vi "WSVCAP SHL Host LL I2C Build and Parse Read Message.vi"(0 "C1 Read Data In":u8[][](array[numeric]) format="%.0x", 1 "Message In":string, 5 "C2 Read Data":u8[][](array[numeric]) format="%.0x", 7 "C3 Read Data":u8[][](array[numeric]) format="%.0x", 9 "Status In":u8[](array[numeric]), 11 "error in":errorcluster) -> (3 "Message Out":string, 4 "C1 Read Data Out":u8[][](array[numeric]) format="%.0x", 6 "C2 Read Data Out":u8[][](array[numeric]) format="%.0x", 8 "C3 Read Data Out":u8[][](array[numeric]) format="%.0x", 10 "Status":u8[](array[numeric]), 15 "error out":errorcluster)   [LabVIEW 2012]
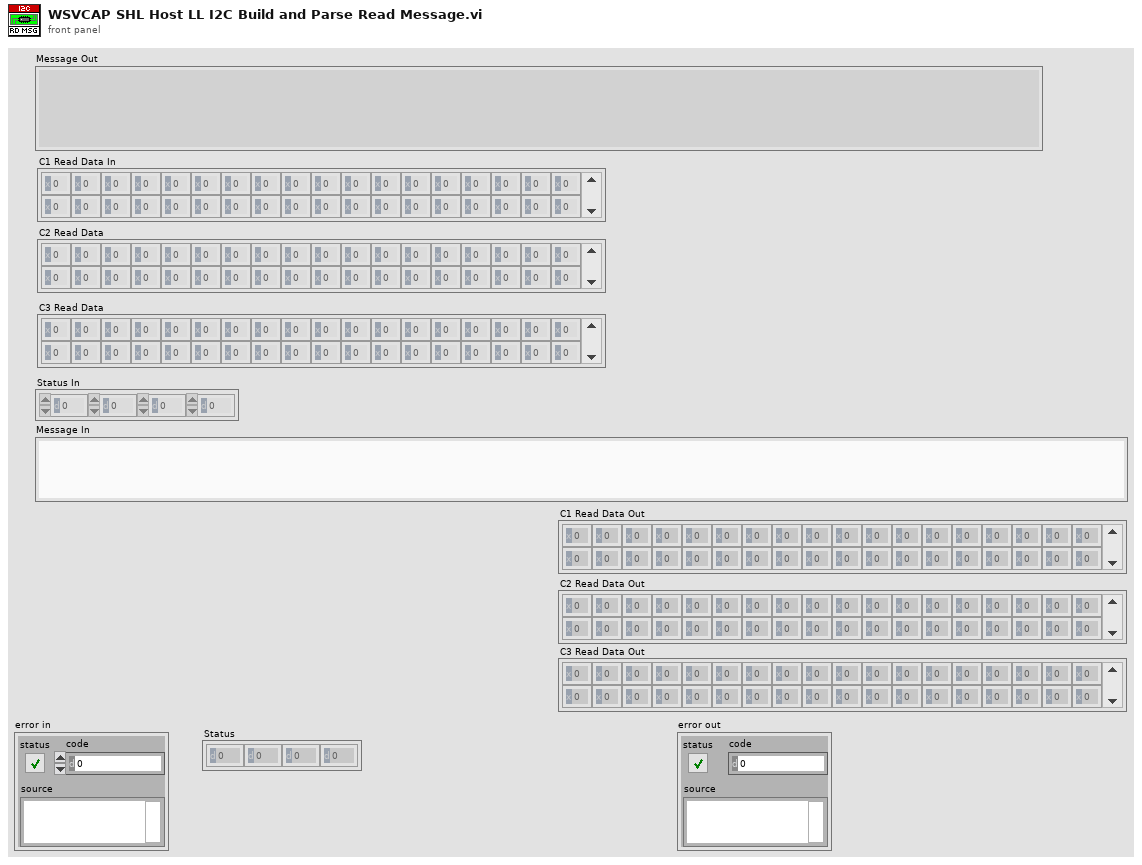
[diagram p1: front panel]
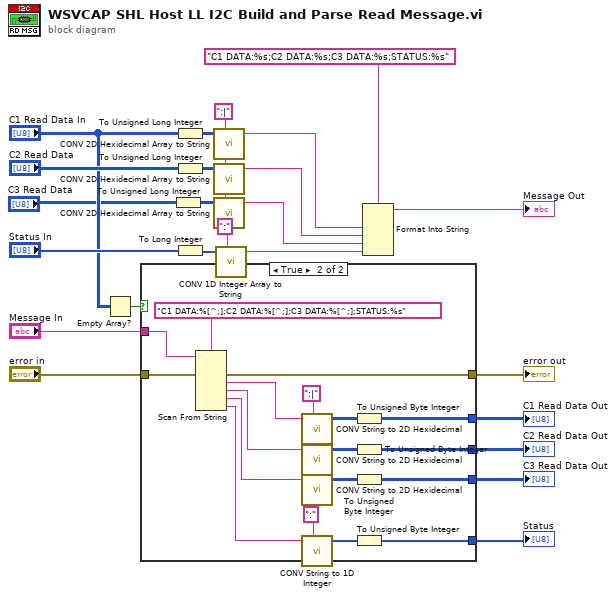
[diagram p0: block diagram]
diagram:
  w4 = ":|" ("Delimiters (,;)")
  n1 = Empty Array?(array="C1 Read Data In") -> (empty?=w8:bool)
  n2 = case shown="True" w8 {
    tunnel: [_ w41] -> w18
    tunnel: [_ w40] -> w17
    tunnel: "error in" -> [w25 w36]
    tunnel: [_ w32] -> w12
    tunnel: "Message In" -> [_ w26]
    tunnel: [w25 w31] -> w7
    tunnel: [_ w27] -> w1
    frame False {
    }
    frame True {
      w28 = ":|" ("Delimiters (,;)")
      n3 = Scan From String(format string="C1 DATA:%[^;];C2 DATA:%[^;];C3 DATA:%[^;];STATUS:%s", input string=w26, error in=w36) -> (error out=w31:errorcluster, output 1=w38:string, output 2=w37:string, output 3=w29:string, output 4=w35:string)  [unwired: 5 in, 2 out]
      n4 = call "CONV String to 2D Hexidecimal.vi"("String"=w38, "Delimiters (,;)"=w28) -> ("2-D Hexidecimal"=w43:u32[][])  [unwired: 7 in]
      n5 = call "CONV String to 2D Hexidecimal.vi"("String"=w37, "Delimiters (,;)"=w28) -> ("2-D Hexidecimal"=w42:u32[][])  [unwired: 7 in]
      n6 = call "CONV String to 2D Hexidecimal.vi"("String"=w29, "Delimiters (,;)"=w28) -> ("2-D Hexidecimal"=w30:u32[][])  [unwired: 7 in]
      n7 = call "CONV String to 1D Integer.vi"("String"=w35, "Delimiter (,)"=":" ("Delimiters (,;)")) -> ("1-D Integer"=w33:i32[])  [unwired: 7 in]
      n8 = To Unsigned Byte Integer(number=w43) -> (unsigned 8bit integer=w41:u8[][])
      n9 = To Unsigned Byte Integer(number=w42) -> (unsigned 8bit integer=w40:u8[][])
      n10 = To Unsigned Byte Integer(number=w30) -> (unsigned 8bit integer=w27:u8[][])
      n11 = To Unsigned Byte Integer(number=w33) -> (unsigned 8bit integer=w32:u8[])
    }
  }
  "C1 Read Data Out" <- w18
  "C2 Read Data Out" <- w17
  "error out" <- w7
  "Status" <- w12
  "C3 Read Data Out" <- w1
  n12 = To Unsigned Long Integer(number="C3 Read Data") -> (unsigned 32bit integer=w6:u32[][])
  n13 = To Unsigned Long Integer(number="C1 Read Data In") -> (unsigned 32bit integer=w24:u32[][])
  n14 = To Unsigned Long Integer(number="C2 Read Data") -> (unsigned 32bit integer=w22:u32[][])
  n15 = To Long Integer(number="Status In") -> (32bit integer=w14:i32[])
  n16 = call "CONV 2D Hexidecimal Array to String.vi"("2-D Hexidecimal"=w24, "Delimiters (,;)"=w4) -> ("String"=w21:string)  [unwired: 7 in]
  n17 = call "CONV 2D Hexidecimal Array to String.vi"("2-D Hexidecimal"=w22, "Delimiters (,;)"=w4) -> ("String"=w20:string)  [unwired: 7 in]
  n18 = call "CONV 2D Hexidecimal Array to String.vi"("2-D Hexidecimal"=w6, "Delimiters (,;)"=w4) -> ("String"=w2:string)  [unwired: 7 in]
  n19 = call "CONV 1D Integer Array to String.vi"("1-D Integer"=w14, "Delimiter (,)"=":" ("Delimiters (,;)")) -> ("String"=w13:string)  [unwired: 7 in]
  n20 = Format Into String(format string="C1 DATA:%s;C2 DATA:%s;C3 DATA:%s;STATUS:%s", w21, w20, w2, w13) -> (resulting string=→"Message Out":string)  [unwired: 2 in, 1 out]
